vi "ReadZ2.vi"() -> ()   [LabVIEW 2022 SP3]
uses:
  <vilib>/Analysis/baseanly.llb/Quick Scale 1D.vi
  <vilib>/Utility/file.llb/Read From Spreadsheet File (string).vi
  <vilib>/Utility/file.llb/Write To Spreadsheet File (DBL).vi
  <vilib>/Analysis/NI_AALBase.lvlib
panel:
  in  "Save Data":bool
  out "output array":dbl[][](array[numeric])
  in  "Ring":u16(ring)
  out "subarray 2":dbl[](array[numeric])
  out "subarray":dbl[](array[numeric])
  out "XY Graph":cluster{dbl[], dbl[]}[](graph)
  in  "Use Selected Files":bool
  in  "Listbox":i32[](listbox)
  in  "Choose Directory":path
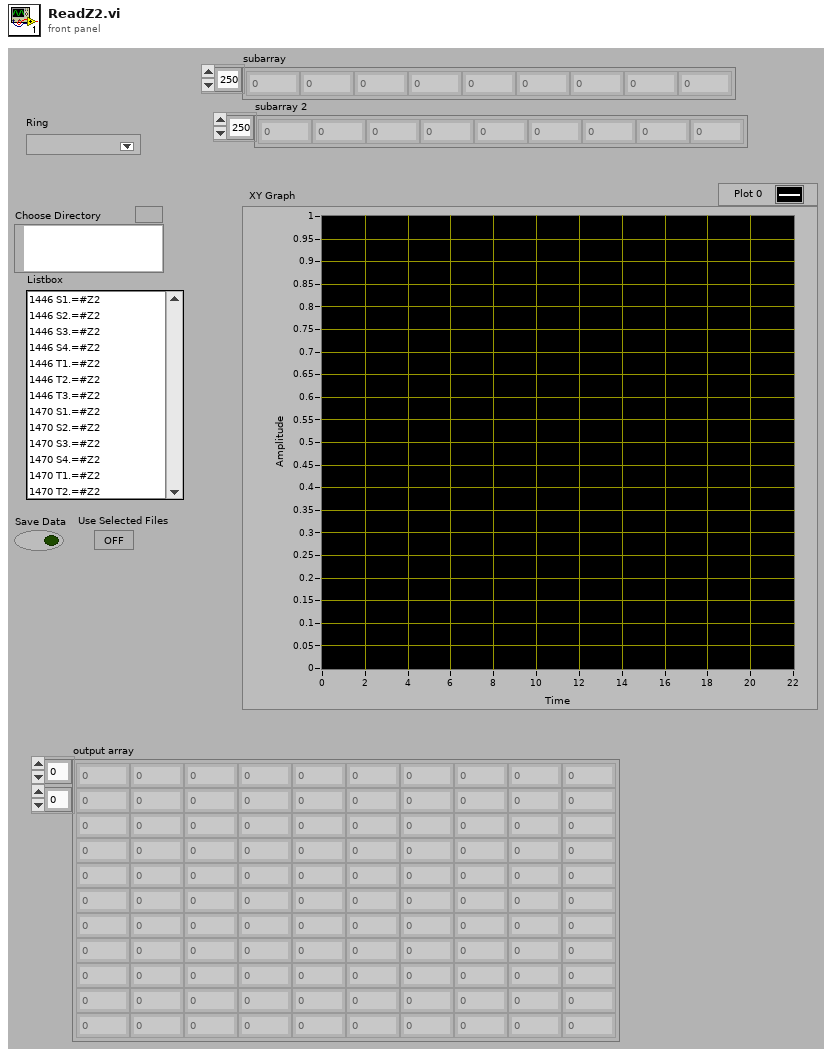
[diagram p1: front panel]
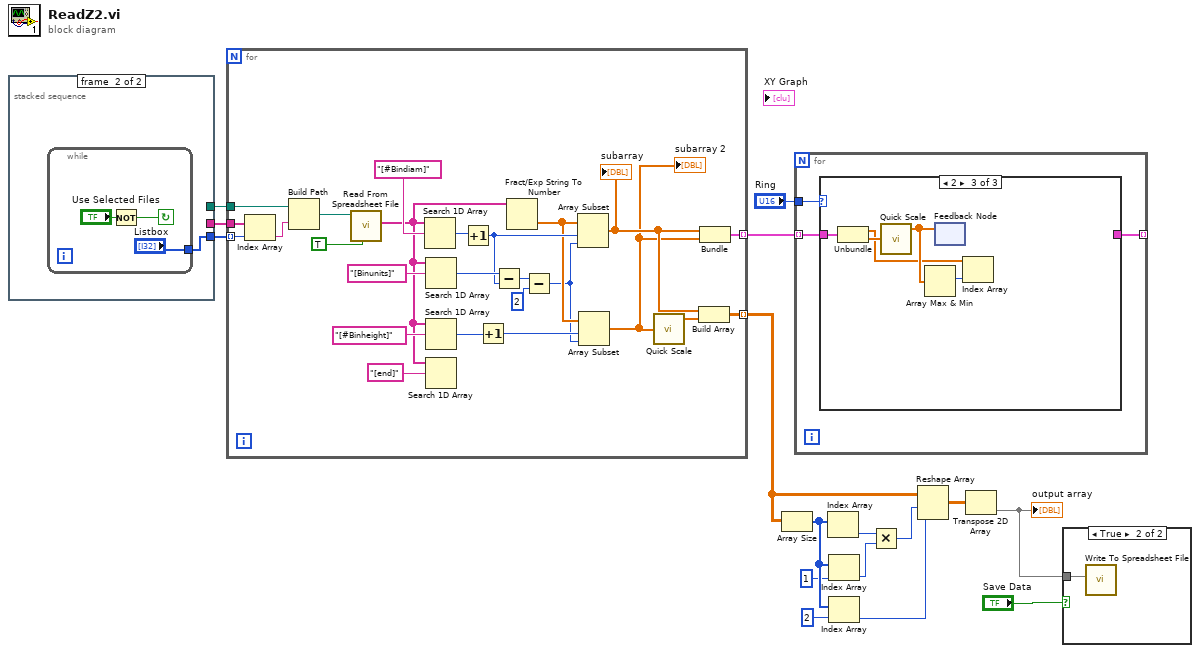
[diagram p0: block diagram]
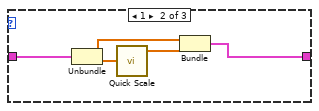
[diagram p4: hidden frame]
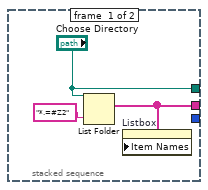
[diagram p5: hidden frame]
diagram:
  n1 = stacked-sequence {
    tunnel: [w18 _] -> w16
    tunnel: [_ w20] -> w15
    tunnel: ["Choose Directory" _] -> w14
    frame #0 {
      n2 = List Folder(path="Choose Directory", pattern="*.=#Z2") -> (filenames=w18:string[])  [unwired: 1 in, 4 out]
      n3 = property on="Listbox" class="LstBox (strict)"("Item Names"=w18) -> ()  [unwired: 2 in, 2 out]
    }
    frame #1 {
      n4 = while {
        tunnel: ["Listbox"] -> w20
        stop <- w22 continue-if-true
        n5 = Not(x="Use Selected Files") -> (.not. x?=w22:bool)
      }
    }
  }
  n6 = for {
    tunnel: w16 -> [w48]
    tunnel: w15 -> [w47] mode=indexing
    tunnel: w14 -> [w45]
    tunnel: [w32] -> w13 mode=indexing
    tunnel: [w26] -> w11 mode=indexing
    n7 = Index Array(array=w48, index=w47) -> (element=w46:string)
    n8 = Build Path(base path=w45, name or relative path=w46) -> (appended path=w44:path)
    n9 = call-poly <vilib>:"Read From Spreadsheet File.vi"("transpose (no:F)"=TRUE, "file path (dialog if empty)"=w44) -> ("first row"=w34:string[])  [unwired: 2 in, 7 out]
    n10 = Search 1D Array(1D array=w34, element="[#Bindiam]") -> (index of element=w39:i32)  [unwired: 1 out]
    n11 = Search 1D Array(1D array=w34, element="[Binunits]") -> (index of element=w37:i32)  [unwired: 1 out]
    n12 = Search 1D Array(1D array=w34, element="[#Binheight]") -> (index of element=w38:i32)  [unwired: 1 out]
    n13 = Search 1D Array(1D array=w34, element="[end]") -> ()  [unwired: 2 out]
    n14 = Increment(x=w39) -> (x+1=w36:i32)
    n15 = Increment(x=w38) -> (x+1=w35:i32)
    n16 = Subtract(x=w37, y=w36) -> (x-y=w29:i32)
    n17 = Fract/Exp String To Number(string=w34) -> (number=w33:dbl[])  [unwired: 4 out]
    n18 = Subtract(x=w29, y=2) -> (x-y=w30:i32)
    n19 = Array Subset(array=w33, index=w36, length=w30) -> (w27:dbl[])
    "subarray" <- w27
    n20 = Array Subset(array=w33, index=w35, length=w30) -> (w25:dbl[])
    "subarray 2" <- w25
    n21 = call-poly <vilib>:"Quick Scale.vi"("X"=w25) -> ("Y[i]=X[i]/Max|X|"=w24:dbl[])  [unwired: 2 out]
    n22 = Build Array(w27, w24) -> (w26:dbl[][])
    n23 = Bundle(w27, w25) -> (w32:cluster{dbl[], dbl[]})  [unwired: 1 out]
  }
  n24 = Array Size(array=w11) -> (size(s)=w10:i32[])
  n25 = for {
    tunnel: w13 -> [w51] mode=indexing
    tunnel: [w50] -> _ mode=indexing
    tunnel: "Ring" -> [w49]
    n26 = case shown="2" w49 {
      tunnel: [w52 w53 _] -> w50
      tunnel: w51 -> [w52 w57 w61]
      frame 0, Default {
      }
      frame 1 {
        n27 = Unbundle(w57) -> (w54:dbl[], w56:dbl[])
        n28 = call-poly <vilib>:"Quick Scale.vi"("X"=w56) -> ("Y[i]=X[i]/Max|X|"=w55:dbl[])  [unwired: 2 out]
        n29 = Bundle(w54, "Y[i]=X[i]/Max|X|"=w55) -> (w53:cluster{dbl[], "Y[i]=X[i]/Max|X|":dbl[]})  [unwired: 1 out]
      }
      frame 2 {
        n30 = Unbundle(w61) -> (w59:dbl[], w62:dbl[])
        n31 = call-poly <vilib>:"Quick Scale.vi"("X"=w62) -> ("Y[i]=X[i]/Max|X|"=w60:dbl[])  [unwired: 2 out]
        n32 = Array Max & Min(array=w60) -> (max index (indices)=w58:i32)  [unwired: 3 out]
        n33 = feedback-in #1(w60) -> ()
        n34 = feedback #1() -> ()  [unwired: 2 out]
        n35 = Index Array(array=w59, index=w58) -> ()  [unwired: 1 out]
      }
    }
  }
  n36 = Index Array(array=w10) -> (element=w7:i32)  [unwired: 1 in]
  n37 = Index Array(array=w10, index=1) -> (element=w6:i32)
  n38 = Index Array(array=w10, index=2) -> (element=w4:i32)
  n39 = Multiply(x=w7, y=w6) -> (x*y=w5:i32)
  n40 = Reshape Array(w11, w5, w4) -> (w3:dbl[][])
  n41 = Transpose 2D Array(2D array=w3) -> (transposed array=w2:dbl[][])
  "output array" <- w2
  n42 = case shown="True" "Save Data" {
    tunnel: w2 -> [_ w63]
    frame False {
    }
    frame True {
      n43 = call-poly <vilib>:"Write To Spreadsheet File.vi"("2D data"=w63) -> ()  [unwired: 5 in, 3 out]
    }
  }
